vi "TEST Move Key.vi"() -> ()   [LabVIEW 2013, in "Carya Config.lvclass"]
doc: "Copyright 2018, Carya Automatisering, Wiebe Walstra."
uses:
  Carya Config.lvclass
panel:
  out "Moved items":i32
  in  "String 2":string="[FilterOptions]\r\nRemove Low Noise=FALSE\r\nApply Thinning=FALSE\r\nApply Envelope=FALSE\r\nThinning - Max distance=10\r\nThinning - Strength=3.000000\r\nLow noise - Filter size=10\r\nLow noise - Transition size=5\r\nApply Interpolation=TRUE\r\n[ImageArea]\r\nis masking enabled=TRUE\r\n[3D Indication]\nY1=103\r\ndY=13\r\nView=1.000000,-0.000000,0.000000,0.000000,0.000000,1.000000,0.000000,0.000000,-0.000000,-0.000000,1.000000,-2.000000,0.000000,0.000000,0.000000,1.000000\r\nComment=interpol.\r\n"
  out "String":string
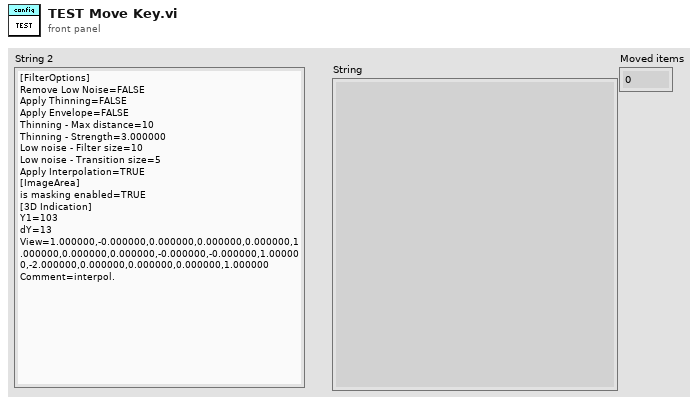
[diagram p1: front panel]
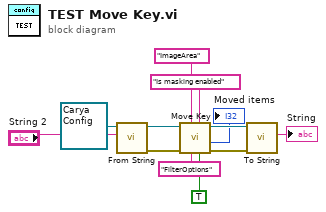
[diagram p0: block diagram]
diagram:
  n1 = call-dynamic "From String.vi"("String"="String 2", "Carya Config in"=refnum<class "Carya Config.lvclass"> refnum) -> ("error out"=w2:errorcluster, "Carya Config out"=w7:refnum<class "Carya Config.lvclass">)  [unwired: 7 in, 1 out]
  n2 = call-dynamic "Move Key.vi"("Overwrite excisting? [F]"=TRUE, "Key name"="Is masking enabled" ("Section name/Regex"), "New section name"="FilterOptions" ("Section name/Regex"), "Section name"="ImageArea" ("Section name/Regex"), "error in (no error)"=w2, "Carya Config in"=w7) -> ("error out"=w1:errorcluster, "Moved items"=→"Moved items":i32, "Carya Config out"=w8:refnum<class "Carya Config.lvclass">)  [unwired: 3 in]
  n3 = call-dynamic "To String.vi"("error in (no error)"=w1, "Carya Config in"=w8) -> ("String"=→"String":string)  [unwired: 7 in, 2 out]
